vi "Write Used Test Numbers.vi"(8 "error in (no error)":errorcluster, 10 "Used Test Numbers":i64[](array[numeric]), 11 "Test Number and Bin Generator in":refnum<class "Test Number and Bin Generator.lvclass">=refnum) -> (0 "error out":errorcluster, 3 "Test Number and Bin Generator out":refnum<class "Test Number and Bin Generator.lvclass">)   [LabVIEW 2018, in "Test Number and Bin Generator.lvlib" / "Test Number and Bin Generator.lvclass"]
uses:
  Test Number and Bin Generator.lvclass
  Test Number and Bin Generator.lvclass/Test Number and Bin Generator.ctl
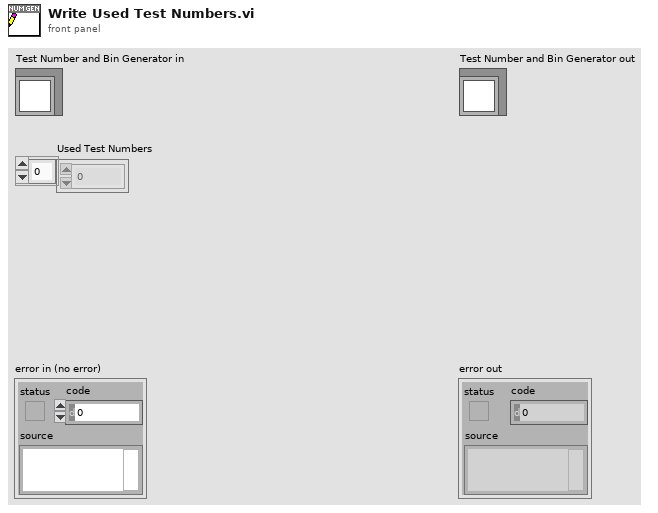
[diagram p1: front panel]
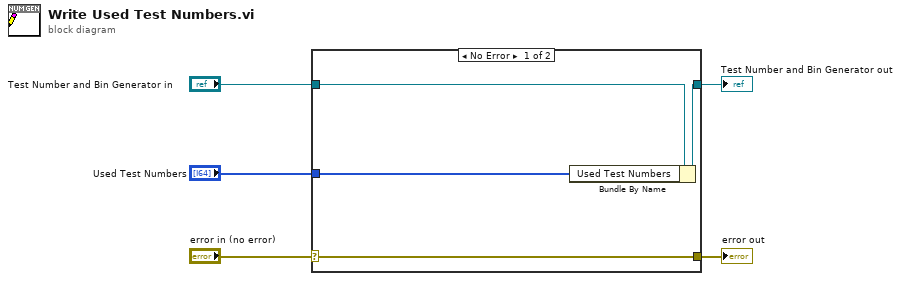
[diagram p0: block diagram]
diagram:
  n1 = case shown="No Error" "error in (no error)" {
    selector: "error in (no error)" -> [w9 w10]
    tunnel: [w9 w10] -> w4
    tunnel: [w7 w11] -> w2
    tunnel: "Test Number and Bin Generator in" -> [w8 w11]
    tunnel: "Used Test Numbers" -> [w6 _]
    frame No Error {
      n2 = Bundle By Name(cluster=w8, "Used Test Numbers"=w6) -> (w7:refnum<class "Test Number and Bin Generator.lvclass">)
    }
    frame Error {
    }
  }
  "error out" <- w4
  "Test Number and Bin Generator out" <- w2
